vi "tcs_getEvent_RejectedCommand.vi"(8 "error in (no error)":errorcluster, 11 "logevent_RejectedCommand_Ctl":T1) -> (0 "error out":errorcluster, 2 "function return":i32, 3 "logevent_RejectedCommand_Ctl out":T1)   [LabVIEW 2016, in "SALLV_tcs.lvlib"]
doc: "int tcs_shm_getEvent_RejectedCommandLV(tcs_logevent_RejectedCommandLV *logevent_RejectedCommand_Ctl );"
uses:
  SALLV_tcs.lvlib
  DataTypes/logevent_RejectedCommand.ctl
  SALLV_tcs.so
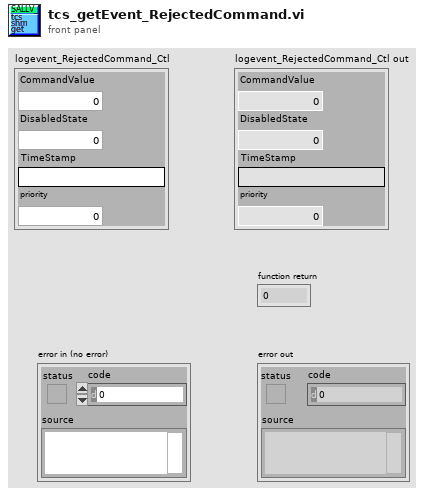
[diagram p1: front panel]
types:
  T1 = typedef "SALLV_tcs.lvlib/logevent_RejectedCommand.ctl" = cluster{"CommandValue":u16, "DisabledState":u16, "TimeStamp":string, "priority":i32}
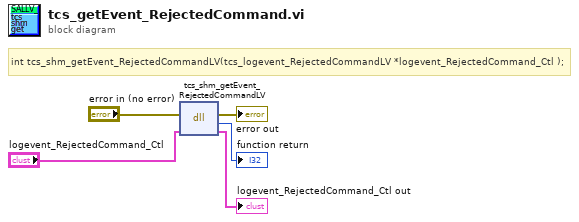
[diagram p0: block diagram]
diagram:
  # "int tcs_shm_getEvent_RejectedCommandLV(tcs_logevent_RejectedCommandLV *logevent_RejectedCommand_Ctl );"
  n1 = dll-call lib="home/saluser/ct_tcs/ts_sallv_tcs/SALLV_tcs.*" fn="tcs_shm_getEvent_RejectedCommandLV"(error in="error in (no error)", "logevent_RejectedCommand_Ctl"="logevent_RejectedCommand_Ctl") -> (error out=→"error out":errorcluster, →"function return":i32, "logevent_RejectedCommand_Ctl"=→"logevent_RejectedCommand_Ctl out":T1)  [unwired: 2 in, 1 out]
